vi "MPPT Real Time.vi"() -> ()   [LabVIEW 2017]
doc: "This example shows how to create, run a script and query the script output data."
uses:
  <instrlib>/Keithley 2600 Series/Keithley 2600 Series.lvlib
panel:
  out "P Vs T":cluster{dbl[], dbl[]}(graph)
  out "Time(Min)":dbl[](array[numeric])
  out "Start Time":string
  out "Iteration No.":i32
  out "Current":dbl[](array[numeric])
  out "P, I Vs V":cluster{dbl[], dbl[]}[](graph)
  out "P(k-1)":dbl
  out "P(k)":dbl
  out "V(k-1)":dbl
  out "V(k)":dbl
  out "Voltage":dbl[](array[numeric])
  out "Power":dbl[](array[numeric])
  in  "Stop":bool
  in  "Delay(s)":u32=15
  in  "dV":dbl=0.01 caption="limitI"
  in  "Initial Voltage (V)":dbl caption="limitI"
  in  "Current Limit (A)":dbl=0.1 caption="limitI"
  in  "USB COM Port":refnum<visa-resource-name>="COM5"
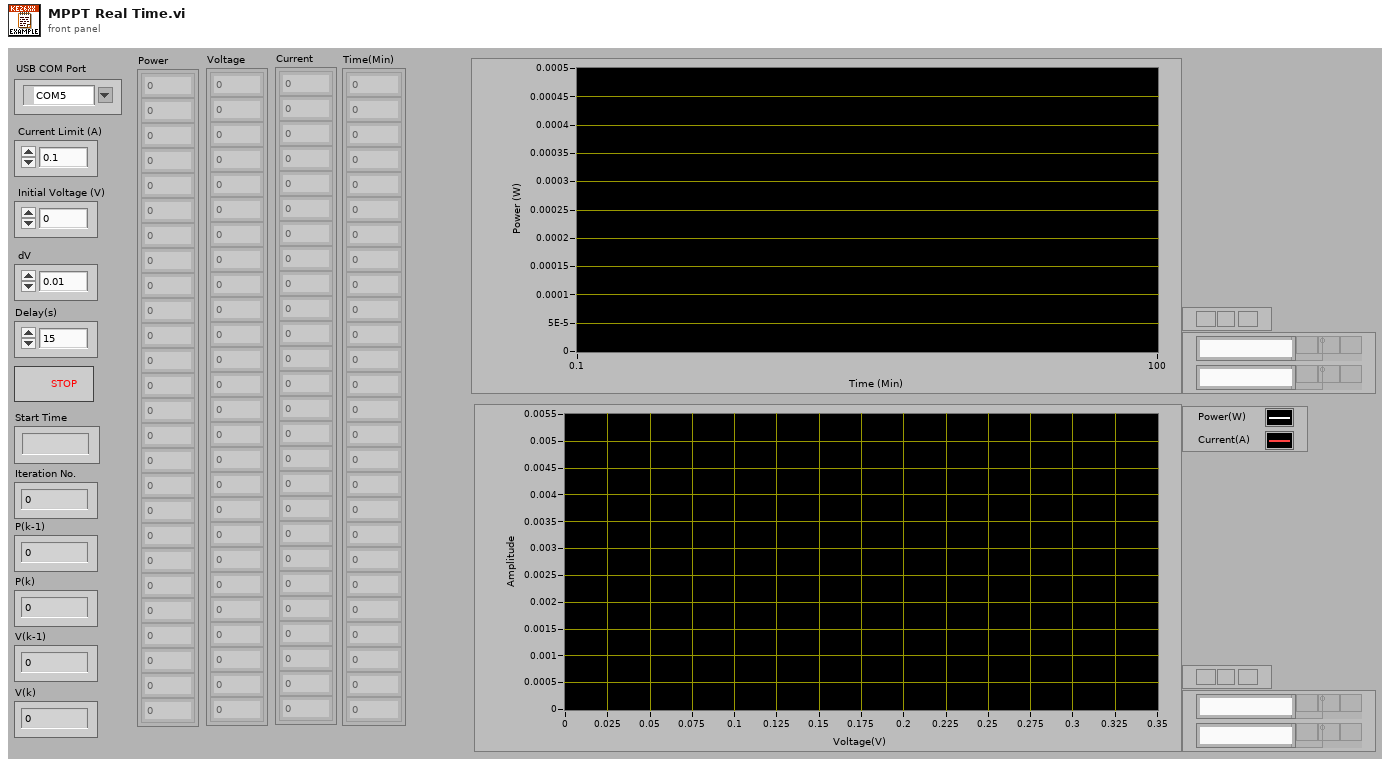
[diagram p1: front panel]
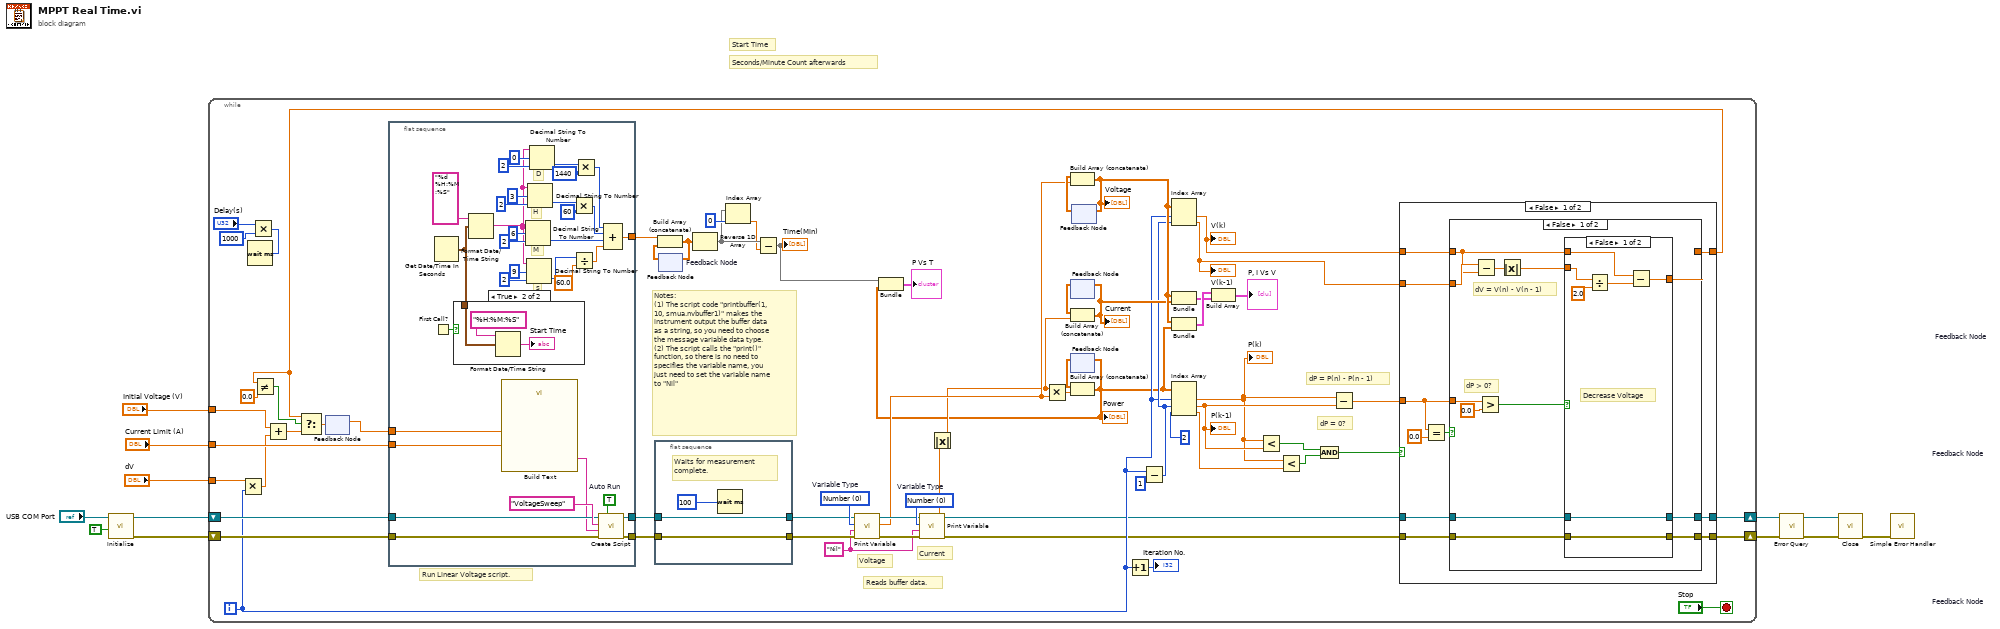
[diagram p0: block diagram]
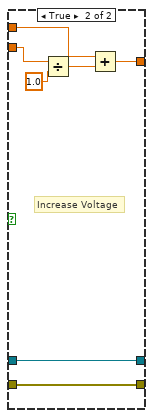
[diagram p2: hidden frame]
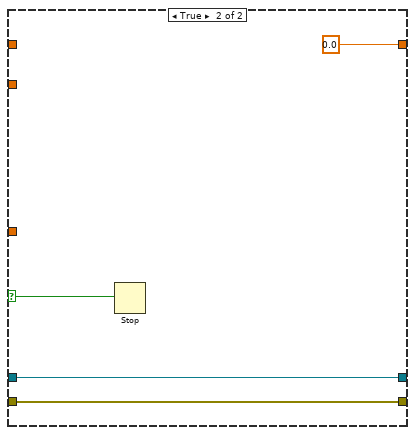
[diagram p4: hidden frame]
diagram:
  # "Seconds/Minute Count afterwards"
  # "Start Time"
  n1 = call <instrlib>:"Initialize.vi"("Reset (True)"=TRUE, "VISA resource name"="USB COM Port") -> ("error out"=w8:errorcluster, "VISA resource name out"=w9:refnum<visa-resource-name>)  [unwired: 8 in]
  n2 = while {
    tunnel: "Current Limit (A)" -> [w66]
    shift-right: [w29] -> w6
    shift-left: w9 -> [w74]
    shift-right: [w28] -> w5
    shift-left: w8 -> [w73]
    tunnel: "dV" -> [w65]
    tunnel: "Initial Voltage (V)" -> [w63]
    i -> [w32]
    stop <- "Stop" stop-if-true
    w62 = "Nil"
    w71 = 0 items=["Number", "Message"]  # Variable Type
    w72 = 0 items=["Number", "Message"]  # Variable Type
    # "dP = 0?"
    # "dP = P(n) - P(n - 1)"
    # "Voltage"
    # "Current"
    # "Reads buffer data."
    # "Notes: \n(1) The script code \"printbuffer(1, 10, smua.nvbuffer1)\" makes the instrument output the buffer data as a string, so you need to choose the message variable data type.\n(2) The script calls the \"print()\" function, so there is no need to specifies the variable name, you just need to set the variable name to \"Nil\""
    # "Run Linear Voltage script."
    n3 = Multiply(x=w65, y=w32) -> (x*y=w64:dbl)
    n4 = Multiply(x="Delay(s)", y=1000) -> (x*y=w24:u32)
    n5 = Wait (ms)(milliseconds to wait=w24) -> ()  [unwired: 1 out]
    n6 = Add(x=w63, y=w64) -> (x+y=w59:dbl)
    n7 = feedback #1() -> (w58:dbl)  [unwired: 1 in]
    n8 = flat-sequence {
      tunnel: [w149] -> w76
      tunnel: [w148] -> w75
      tunnel: w74 -> [w147]
      tunnel: w73 -> [w146]
      tunnel: w66 -> [w144]
      tunnel: w58 -> [w143]
      tunnel: [w120] -> w17
      frame #0 {
        w150 = TRUE  # Auto Run
        # "D"
        # "H"
        # "M"
        # "S"
        n9 = First Call?() -> (First Call?: T/F=w121:bool)
        n10 = Get Date/Time In Seconds() -> (seconds since 1Jan1904=w122:timestamp)
        n11 = case shown="True" w121 {
          tunnel: w122 -> [_ w153]
          frame False {
          }
          frame True {
            n12 = Format Date/Time String(time format string (%c)="%H:%M:%S", seconds (now)=w153) -> (date/time string=→"Start Time":string)  [unwired: 1 out]
          }
        }
        n13 = Format Date/Time String(time format string (%c)="%d %H:%M:%S", seconds (now)=w122) -> (date/time string=w125:string)  [unwired: 1 out]
        n14 = call "Build Text"("limitI"=w144, "volt"=w143) -> ("Result"=w145:string)  [unwired: 12 in, 1 out]
        n15 = Decimal String To Number(string=w125, offset=6 ("offset (0)"), default (0L)=2 ("length (rest)")) -> (number=w135:i32)  [unwired: 1 out]
        n16 = Decimal String To Number(string=w125, offset=9 ("offset (0)"), default (0L)=2 ("length (rest)")) -> (number=w134:i32)  [unwired: 1 out]
        n17 = Decimal String To Number(string=w125, offset=3 ("offset (0)"), default (0L)=2 ("length (rest)")) -> (number=w131:i32)  [unwired: 1 out]
        n18 = Decimal String To Number(string=w125, offset=0 ("offset (0)"), default (0L)=2 ("length (rest)")) -> (number=w128:i32)  [unwired: 1 out]
        n19 = Multiply(x=w131, y=60) -> (x*y=w132:i32)
        n20 = Divide(x=w134, y=60.0) -> (x/y=w133:dbl)
        n21 = Multiply(x=w128, y=1440) -> (x*y=w124:i32)
        n22 = call <instrlib>:"Create Script.vi"("Auto Run (F: Disable)"=w150, "error in (no error)"=w146, "Source Code"=w145, "Script Variable"="VoltageSweep" ("Script Variable (myScript)"), "VISA resource name"=w147) -> ("error out"=w148:errorcluster, "VISA resource name out"=w149:refnum<visa-resource-name>)  [unwired: 5 in]
        n23 = Compound Arithmetic op=ADD(w124, w132, w135, w133) -> (w120:dbl)
      }
    }
    n24 = flat-sequence {
      tunnel: w76 -> [w155]
      tunnel: w75 -> [w156]
      tunnel: [w156] -> w67
      tunnel: [w155] -> w68
      frame #0 {
        # "Waits for measurement complete."
        n25 = Wait (ms)(milliseconds to wait=100 ("Temp Delay")) -> ()  [unwired: 1 out]
      }
    }
    n26 = feedback #2 "Feedback Node"() -> (w22:dbl[])  [unwired: 1 in]
    n27 = Build Array (concatenate)(w17, w22) -> (w21:dbl[])
    n28 = feedback-in #2(w21) -> ()
    n29 = Reverse 1D Array(array=w21) -> (reversed array=w19:dbl[])
    n30 = Index Array(array=w19, index=0) -> (element=w18:dbl)
    n31 = Subtract(x=w19, y=w18) -> (x-y=w15:dbl[])
    "Time(Min)" <- w15
    n32 = call <instrlib>:"Print Variable.vi"("error in (no error)"=w67, "Variable Name"=w62, "Variable Type (0: Number)"=w72, "VISA resource name"=w68) -> ("error out"=w69:errorcluster, "Number"=w33:dbl, "VISA resource name out"=w70:refnum<visa-resource-name>)  [unwired: 4 in, 1 out]
    n33 = call <instrlib>:"Print Variable.vi"("error in (no error)"=w69, "Variable Name"=w62, "Variable Type (0: Number)"=w71, "VISA resource name"=w70) -> ("error out"=w30:errorcluster, "Number"=w26:dbl, "VISA resource name out"=w31:refnum<visa-resource-name>)  [unwired: 4 in, 1 out]
    n34 = Absolute Value(x=w26) -> (abs(x)=w25:dbl)
    n35 = Multiply(x=w25, y=w33) -> (x*y=w53:dbl)
    n36 = feedback #3 "Feedback Node"() -> (w52:dbl[])  [unwired: 1 in]
    n37 = Build Array (concatenate)(w52, w25) -> (w46:dbl[])
    "Current" <- w46
    n38 = feedback-in #3(w46) -> ()
    n39 = feedback #4 "Feedback Node"() -> (w54:dbl[])  [unwired: 1 in]
    n40 = Build Array (concatenate)(w54, w53) -> (w14:dbl[])
    "Power" <- w14
    n41 = Bundle(w15, w14) -> (→"P Vs T":cluster{dbl[], dbl[]})  [unwired: 1 in]
    n42 = feedback-in #4(w14) -> ()
    n43 = feedback #5 "Feedback Node"() -> (w51:dbl[])  [unwired: 1 in]
    n44 = Build Array (concatenate)(w51, w33) -> (w50:dbl[])
    "Voltage" <- w50
    n45 = feedback-in #5(w50) -> ()
    n46 = Increment(x=w32) -> (x+1=→"Iteration No.":i32)
    n47 = Subtract(x=w32, y=1) -> (x-y=w44:i32)
    n48 = Index Array(array=w50, index #1=w32, index #2=w44) -> (element #1=w43:dbl, element #2=w34:dbl)
    "V(k)" <- w43
    "V(k-1)" <- w34
    n49 = Bundle(w50, w46) -> (w48:cluster{dbl[], dbl[]})  [unwired: 1 in]
    n50 = Bundle(w50, w14) -> (w49:cluster{dbl[], dbl[]})  [unwired: 1 in]
    n51 = Index Array(array=w14, index #1=w32, index #2=w44, index #3=2 ("index")) -> (element #1=w37:dbl, element #2=w41:dbl, element #3=w36:dbl)
    "P(k)" <- w37
    "P(k-1)" <- w41
    n52 = Build Array(w49, w48) -> (→"P, I Vs V":cluster{dbl[], dbl[]}[])
    n53 = Less?(x=w37, y=w41) -> (x < y?=w39:bool)
    n54 = Less?(x=w37, y=w36) -> (x < y?=w38:bool)
    n55 = And(x=w39, y=w38) -> (x .and. y?=w40:bool)
    n56 = Subtract(x=w37, y=w41) -> (x-y=w42:dbl)
    n57 = case shown="False" w40 {
      selector: w40 -> [_ w118]
      tunnel: w43 -> [w86 _]
      tunnel: w34 -> [w85 _]
      tunnel: w42 -> [w82 _]
      tunnel: [w84 0.0] -> w27
      tunnel: w31 -> [w80 w117]
      tunnel: w30 -> [w79 w116]
      tunnel: [w78 w117] -> w29
      tunnel: [w77 w116] -> w28
      frame False {
        n58 = Equal?(x=w82, y=0.0) -> (x = y?=w81:bool)
        n59 = case shown="False" w81 {
          tunnel: w86 -> [w91 w115]
          tunnel: w85 -> [w94 _]
          tunnel: [w95 w115] -> w84
          tunnel: w82 -> [w96 _]
          tunnel: w80 -> [w89 w114]
          tunnel: w79 -> [w90 w113]
          tunnel: [w88 w114] -> w78
          tunnel: [w87 w113] -> w77
          frame False {
            # "dV = V(n) - V(n - 1)"
            # "dP > 0?"
            n60 = Subtract(x=w94, y=w91) -> (x-y=w93:dbl)
            n61 = Greater?(x=w96, y=0.0) -> (0:w97:bool)
            n62 = Absolute Value(x=w93) -> (abs(x)=w92:dbl)
            n63 = case shown="False" w97 {
              tunnel: [w103 w110] -> w95
              tunnel: w92 -> [w105 w111]
              tunnel: w91 -> [w104 w112]
              tunnel: w90 -> [w99 w106]
              tunnel: w89 -> [w100 w107]
              tunnel: [w100 w107] -> w88
              tunnel: [w99 w106] -> w87
              frame False {
                # "Decrease Voltage"
                n64 = Divide(x=w105, y=2.0) -> (x/y=w102:dbl)
                n65 = Subtract(x=w104, y=w102) -> (x-y=w103:dbl)
              }
              frame True {
                # "Increase Voltage"
                n66 = Divide(x=w111, y=1.0) -> (x/y=w109:dbl)
                n67 = Add(x=w112, y=w109) -> (x+y=w110:dbl)
              }
            }
          }
          frame True {
          }
        }
      }
      frame True {
        n68 = Stop(stop? (T)=w118) -> ()
      }
    }
    n69 = Not Equal?(x=w27, y=0.0) -> (x != y?=w57:bool)
    n70 = Select(t=w27, s=w57, f=w59) -> (s? t:f=w60:dbl)
    n71 = feedback-in #1(w60) -> ()
  }
  n72 = call <instrlib>:"Error Query.vi"("error in (no error)"=w5, "VISA resource name"=w6) -> ("error out"=w11:errorcluster, "VISA resource name out"=w12:refnum<visa-resource-name>)  [unwired: 6 in, 2 out]
  n73 = call <instrlib>:"Close.vi"("error in (no error)"=w11, "VISA resource name"=w12) -> ("error out"=w1:errorcluster)  [unwired: 9 in]
  n74 = call <vilib>:"Simple Error Handler.vi"("error in (no error)"=w1) -> ()  [unwired: 4 in, 5 out]
